vi "Get Owning Path Default Value.vi"(0 "SG SC2250 Path Group in":refnum<class "SG SC2250 Path Group.lvclass">, 11 "error in (no error)":errorcluster) -> (4 "SG SC2250 Path Group out":refnum<class "SG SC2250 Path Group.lvclass">, 6 "Calibration Common.lvlib:Path.lvclass":refnum<class "Path.lvclass">, 15 "error out":errorcluster)   [LabVIEW 2023, in "RFFixtureCharact.RFPM.lvlib" / "SG SC2250 Path Group.lvclass"]
uses:
  SG SC2250 Path Group.lvclass
  Common/Base Classes/Path/Path.lvclass
  Paths/SG SC2250 Path/SG SC2250 Path.lvclass
  C:/srd-semi-rfcal-software/AuxTools/STSRFFixtureCharactUtility/Source/Code Modules/Common/Base Classes/Path/Path.lvclass
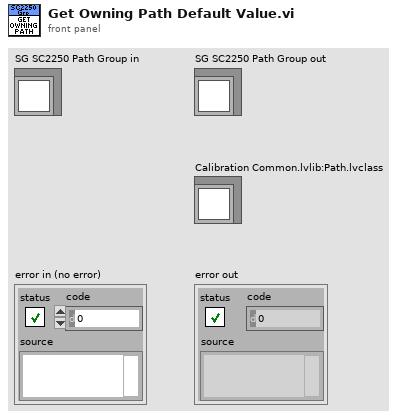
[diagram p1: front panel]
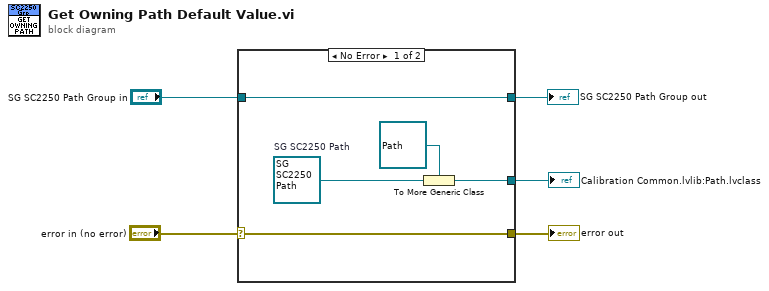
[diagram p0: block diagram]
diagram:
  n1 = case shown="No Error" "error in (no error)" {
    selector: "error in (no error)" -> [w7 w11]
    tunnel: [w8 _] -> w5
    tunnel: [w7 w11] -> w3
    tunnel: [w6 w12] -> w2
    tunnel: "SG SC2250 Path Group in" -> [w6 w12]
    frame No Error {
      w9 = refnum<class "SG SC2250 Path.lvclass"> refnum  # SG SC2250 Path
      n2 = To More Generic Class(target class=refnum<class "Path.lvclass"> refnum ("Path"), reference=w9) -> (generic class reference=w8:refnum<class "Path.lvclass">)
    }
    frame Error {
    }
  }
  "error out" <- w3
  "SG SC2250 Path Group out" <- w2
  "Calibration Common.lvlib:Path.lvclass" <- w5
